vi "testOptimization.vi"() -> ()   [LabVIEW 2017]
uses:
  Adder/Adder0/Adder0.lvclass
  C:/PowerElectronicControl/NonreentrantSinglePoint/dev/Adder/Adder.lvclass
  Subtractor/Subtractor0/Subtractor0.lvclass
  C:/PowerElectronicControl/NonreentrantSinglePoint/dev/Subtractor/Subtractor.lvclass
  Multiplier/Multiply0/Multiplier0.lvclass
  C:/PowerElectronicControl/NonreentrantSinglePoint/dev/Multiplier/Multiplier.lvclass
  Adder/Adder.lvclass
  Multiplier/Multiplier.lvclass
  Subtractor/Subtractor.lvclass
  <vilib>/rvi/Emulation/niFpgaGetClockAttributes.vi
  <vilib>/rvi/Emulation/niFpgaSctlEmulationGetInTimedLoop.vi
  <vilib>/rvi/Emulation/niFpgaEmulationReportErrorSimple.vi
  <vilib>/rvi/Emulation/niFpgaCriticalErrorInLSC.vi
panel:
  out "rate":u32
  in  "C":sgl
  in  "B":sgl
  in  "A":sgl
  out "beta":sgl
  out "alpha":sgl
  in  "C 2":sgl
  in  "B 2":sgl
  in  "A 2":sgl
  out "beta 2":sgl
  out "alpha 2":sgl
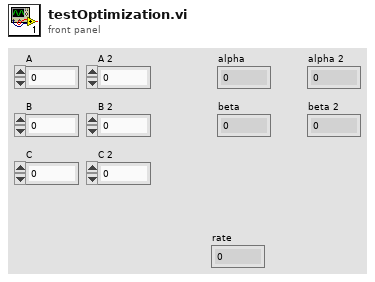
[diagram p1: front panel]
types:
  T1 = cluster{"Adder":refnum<class "Adder.lvclass">, "Multiplier":refnum<class "Multiplier.lvclass">, "Subtractor":refnum<class "Subtractor.lvclass">}
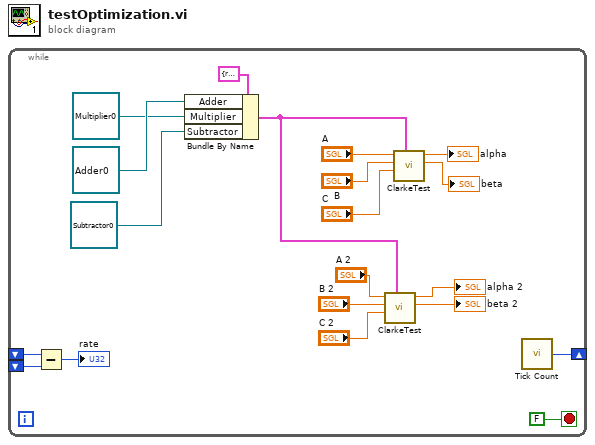
[diagram p0: block diagram]
diagram:
  n1 = while {
    shift-right: [w19] -> _
    shift-left: _ -> [w17]
    shift-left: _ -> [w18]
    stop <- FALSE stop-if-true
    n2 = Subtract(x=w17, y=w18) -> (x-y=→"rate":u32)
    n3 = Bundle By Name(cluster=T1 {"Adder"=refnum, "Multiplier"=refnum, "Subtractor"=refnum} ("Resources"), "Adder"=refnum<class "Adder0.lvclass"> refnum ("Adder0.lvclass"), "Multiplier"=refnum<class "Multiplier0.lvclass"> refnum ("Multiplier0.lvclass"), "Subtractor"=refnum<class "Subtractor0.lvclass"> refnum ("Subtractor0.lvclass")) -> (w1:T1)
    n4 = call "ClarkeTest.vi"("Resources"=w1, "C"="C 2", "B"="B 2", "A"="A 2") -> ("beta"=→"beta 2":sgl, "alpha"=→"alpha 2":sgl)  [unwired: 6 in]
    n5 = call "ClarkeTest.vi"("Resources"=w1, "C"="C", "B"="B", "A"="A") -> ("beta"=→"beta":sgl, "alpha"=→"alpha":sgl)  [unwired: 6 in]
    n6 = call "Tick Count"() -> ("Tick Count(Ticks)"=w19:u32)
  }
